vi "ObjectsMeasurmentsToArray-1.vi"(1 "[IN] Particle Reports (Pixels)":T1(array[cluster]) {"Orientation" format="%.2f"; "Dimensions"."Height" format="%.2f"; "Dimensions"."Width" format="%.2f"; "Center of Mass"."Y" format="%.2f"; "Center of Mass"."X" format="%.2f"; "Bounding Rect"."Bottom" format="%.2f"; "Bounding Rect"."Right" format="%.2f"; "Bounding Rect"."Top" format="%.2f"; "Bounding Rect"."Left" format="%.2f"; "Number of Holes" format="%.2f"; "Area" format="%.2f"}) -> (0 "[OUT] X,Y Coordinates":dbl[](array[numeric]))   [LabVIEW 2020]
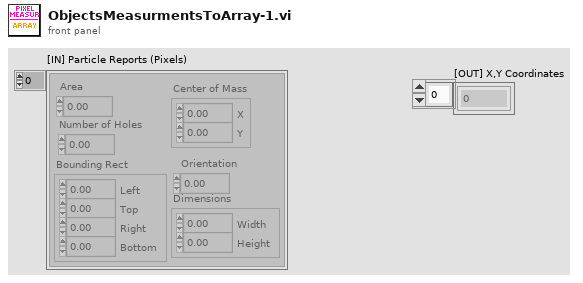
[diagram p1: front panel]
types:
  T1 = cluster{"Area":dbl, "Number of Holes":dbl, "Bounding Rect":cluster{"Left":dbl, "Top":dbl, "Right":dbl, "Bottom":dbl}, "Center of Mass":cluster{"X":dbl, "Y":dbl}, "Orientation":dbl, "Dimensions":cluster{"Width":dbl, "Height":dbl}}[]
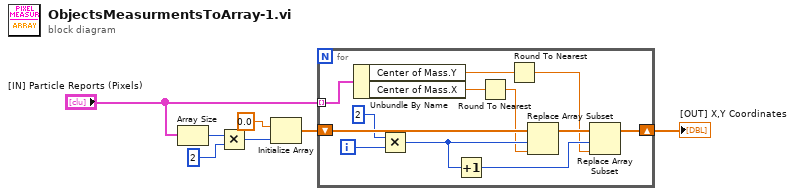
[diagram p0: block diagram]
diagram:
  n1 = Array Size(array="[IN] Particle Reports (Pixels)") -> (size(s)=w6:i32)
  n2 = Multiply(x=w6, y=2) -> (x*y=w4:i32)
  n3 = Initialize Array(0.0 ("element"), w4) -> (w3:dbl[])
  n4 = for {
    tunnel: "[IN] Particle Reports (Pixels)" -> [w19] mode=indexing
    shift-right: [w12] -> w2
    shift-left: w3 -> [w18]
    i -> [w17]
    n5 = Unbundle By Name(w19) -> ("Center of Mass.Y"=w11:dbl, "Center of Mass.X"=w10:dbl)
    n6 = Multiply(x=2 ("y"), y=w17) -> (x*y=w15:i32)
    n7 = Increment(x=w15) -> (x+1=w13:i32)
    n8 = Round To Nearest(number=w10) -> (nearest integer value=w9:dbl)
    n9 = Round To Nearest(number=w11) -> (nearest integer value=w8:dbl)
    n10 = Replace Array Subset(array=w18, new element=w9, index=w15) -> (w14:dbl[])
    n11 = Replace Array Subset(array=w14, new element=w8, index=w13) -> (w12:dbl[])
  }
  "[OUT] X,Y Coordinates" <- w2
